vi "Keithley DMM7510 Acquire Single.vi"(7 "Function":u16(ring) items=["Voltage: DC", "Voltage: AC", "Current: DC", "Current: AC", "2W Resistance", "4W Resistance", "Diode", "Capacitance", "Temperature", "Continuity", "Frequency", "Period", "Ratio", "Digitize Voltage", "Digitize Current"], 8 "error in (no error)":errorcluster, 11 "VISA resource name":refnum<visa-resource-name>) -> (0 "error out":errorcluster caption="错误输出", 3 "Measurement":dbl format="%#_8g")   [LabVIEW 2015]
doc: "This example shows how to configure a measurement and take a reading."
uses:
  Keithley DMM7510.lvlib
panel:
  # "(c) 2015 Keithley Instruments,  ALL RIGHTS RESERVED."
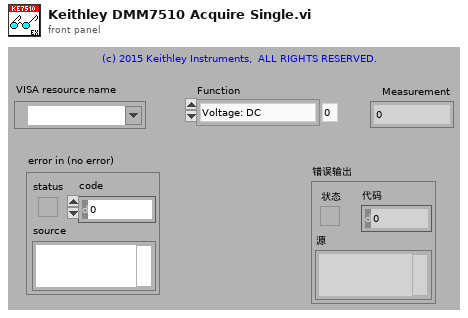
[diagram p1: front panel]
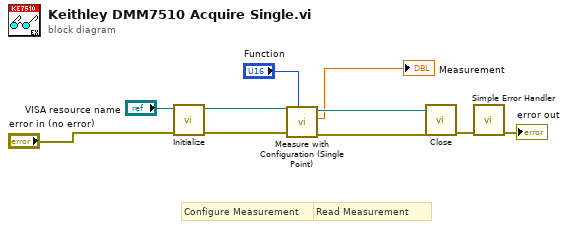
[diagram p0: block diagram]
diagram:
  # "Read Measurement"
  # "Configure Measurement"
  n1 = call "Initialize.vi"("error in (no error)"="error in (no error)", "VISA resource name"="VISA resource name") -> ("error out"=w3:errorcluster, "VISA resource name out"=w8:refnum<visa-resource-name>)  [unwired: 8 in]
  n2 = call "Measure with Configuration (Single Point).vi"("Function"="Function", "error in (no error)"=w3, "VISA resource name"=w8) -> ("error out"=w6:errorcluster, "Measurement"=→"Measurement":dbl, "VISA resource name out"=w7:refnum<visa-resource-name>)  [unwired: 5 in, 1 out]
  n3 = call "Close.vi"("error in (no error)"=w6, "VISA resource name"=w7) -> ("error out"=w10:errorcluster)  [unwired: 9 in]
  n4 = call <vilib>:"Simple Error Handler.vi"("error in (no error)"=w10) -> ("error out"=→"error out":errorcluster)  [unwired: 4 in, 4 out]
